vi "MMB SubVI.vi"(3 "Mode":T1(ring), 4 "Array Size":T2={"Width"=60, "Height"=17}, 5 "LED Off Color":u32(colorbox), 6 "LED Size":T2={"Width"=17, "Height"=17}, 7 "LED On Color":u32(colorbox)=4914962, 8 "Repeat/Hold":u64=1 min=1 step=1, 9 "Delay":u32(knob)=50 scale=0.0..1000.0, 10 "Message":string="The Quick Brown Fox Jumped Over the Lazy Dog", 11 "Config Path":path=path "c:/Ed's Files/LabVIEW Files/Moving Message Board/mmb.ini") -> ()   [LabVIEW 2010]
doc: "INTRODUCTION:\nThis program is a subVI implementation of the Moving Message Board program. It simulates a moving message board made up of an array of LED's or lights. It has multiple modes of operation.\n\nREQUIREMENTS:\nThe calling VI should pass the following inputs to it: the path of the configuration file, a string with the message to be displayed, an integer with the delay time, an integer with the repeat or hold value, and an enum with the operating mode.\n\nOPTIONAL:\nThe following can be passed if desired, but this is not required: a cluster with the \"on\" color of the LED's in the display, a cluster with the \"off\" color of the LED's in the display, a cluster containing the LED width and height, and a cluster containing the display size width and height (based on number of LED's in the array)."
uses:
  <vilib>/Utility/miscctls.llb/LVBoundsTypeDef.ctl
  <vilib>/Utility/miscctls.llb/LVPointTypeDef.ctl
  <vilib>/Utility/config.llb/Read Key (I32).vi
  <userlib>/_OpenG.lib/array/array.llb/Reorder 2D Array2 (Boolean)__ogtk.vi
  <vilib>/Utility/config.llb/NI_LVConfig.lvlib
panel:
  out "Array":bool[][](array[boolean])
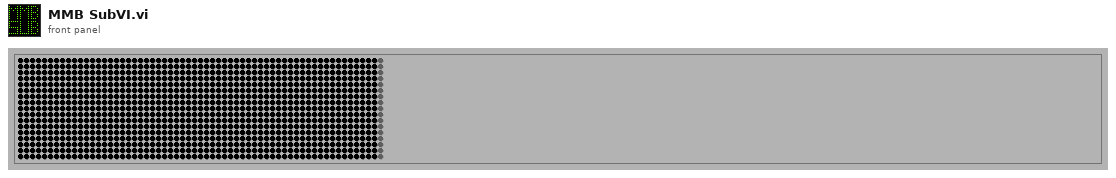
[diagram p1: front panel]
types:
  T1 = enum16{"Scrolling Message (0)", "Non-Scrolling Message (1)", "Fade In (2)", "Fade Out (3)", "Blink (4)", "Fly Up (5)", "Fall Down (6)", "Dissolve In (7)", "Dissolve Out (8)", "Random Pattern (9)"}
  T2 = typedef "LVBoundsTypeDef.ctl" = cluster{"Width":u32, "Height":u32}
  T3 = typedef "LVPointTypeDef.ctl" = cluster{"Horizontal":i16, "Vertical":i16}
  T4 = cluster{"LED Off Color":u32, "LED Off Color":u32}
  T5 = cluster{"LED On Color":u32, "LED On Color":u32}[]
  T6 = typedef "NI_LVConfig.lvlib/Config Data RefNum.ctl" = refnum<k1>
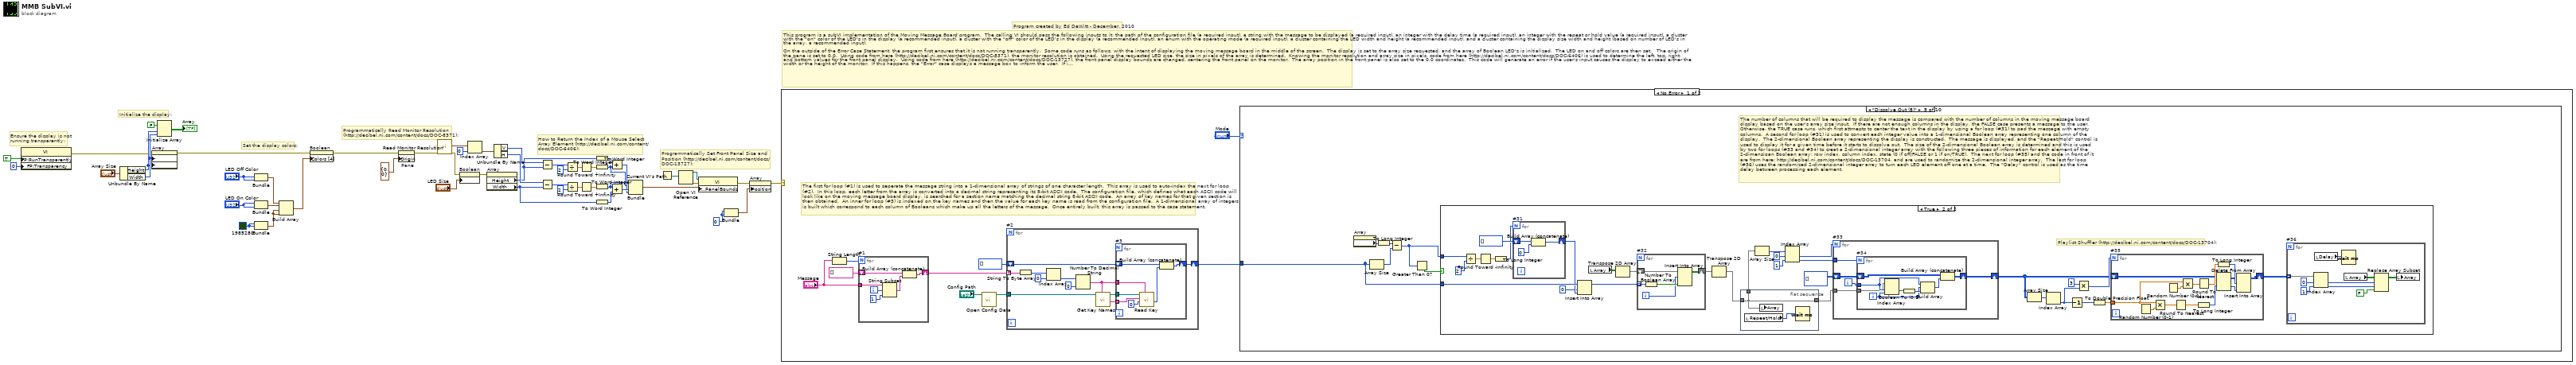
[diagram p0: block diagram]
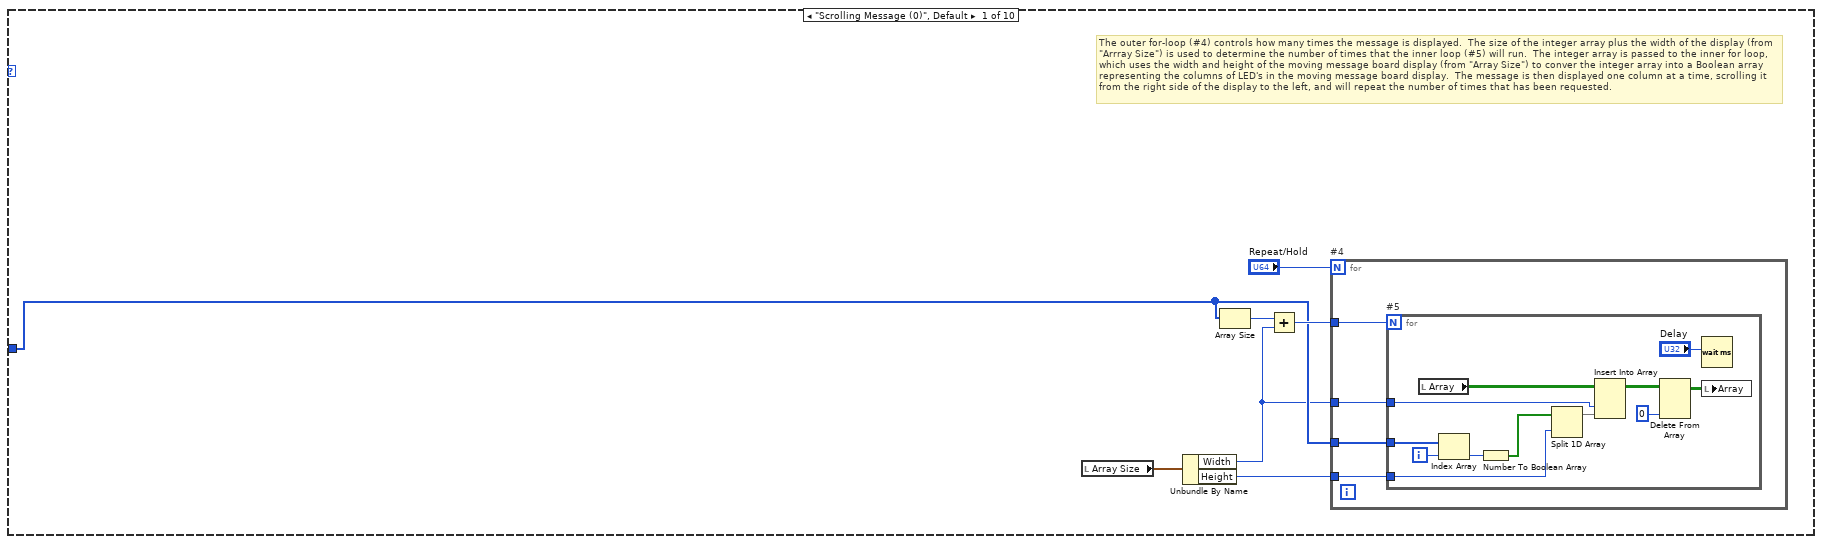
[diagram p2: hidden frame]
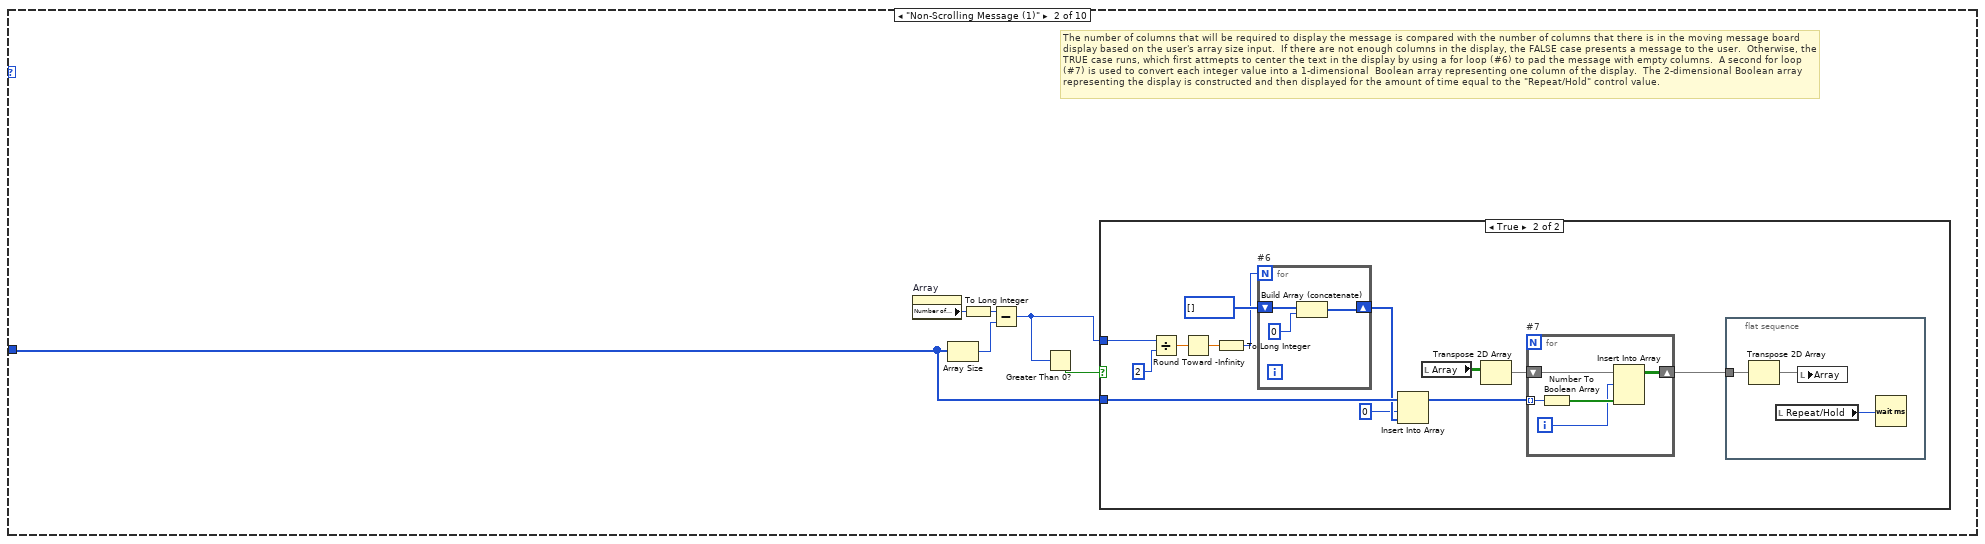
[diagram p3: hidden frame]
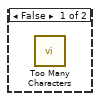
[diagram p4: hidden frame]
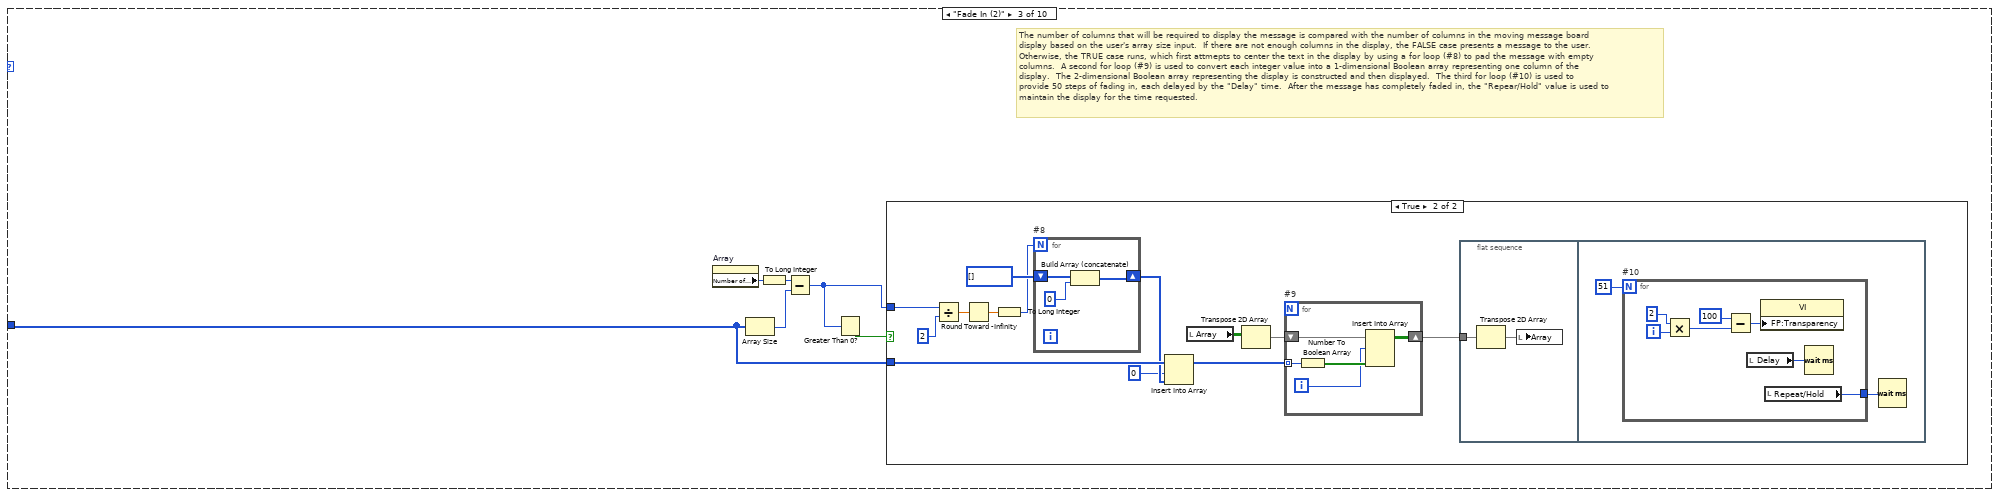
[diagram p5: hidden frame]
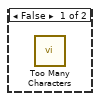
[diagram p6: hidden frame]
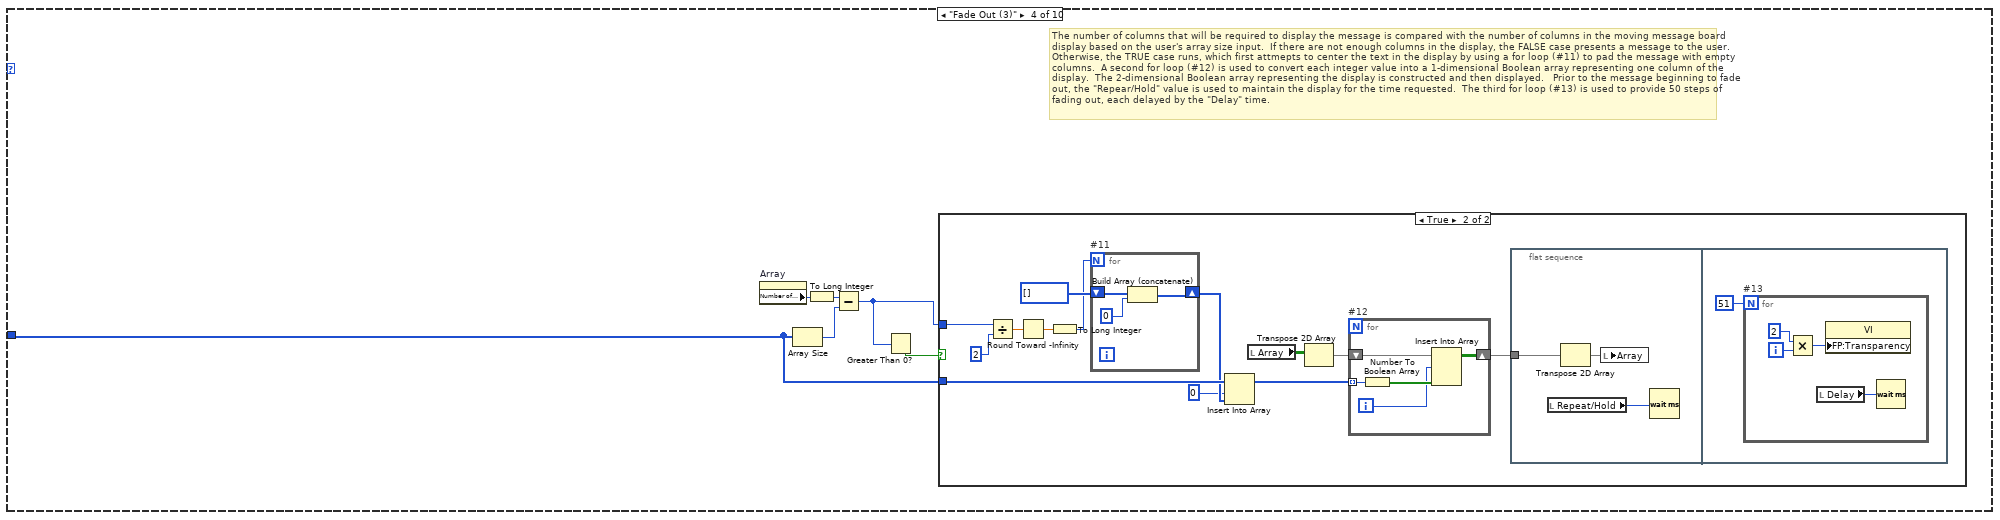
[diagram p7: hidden frame]
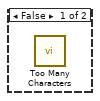
[diagram p8: hidden frame]
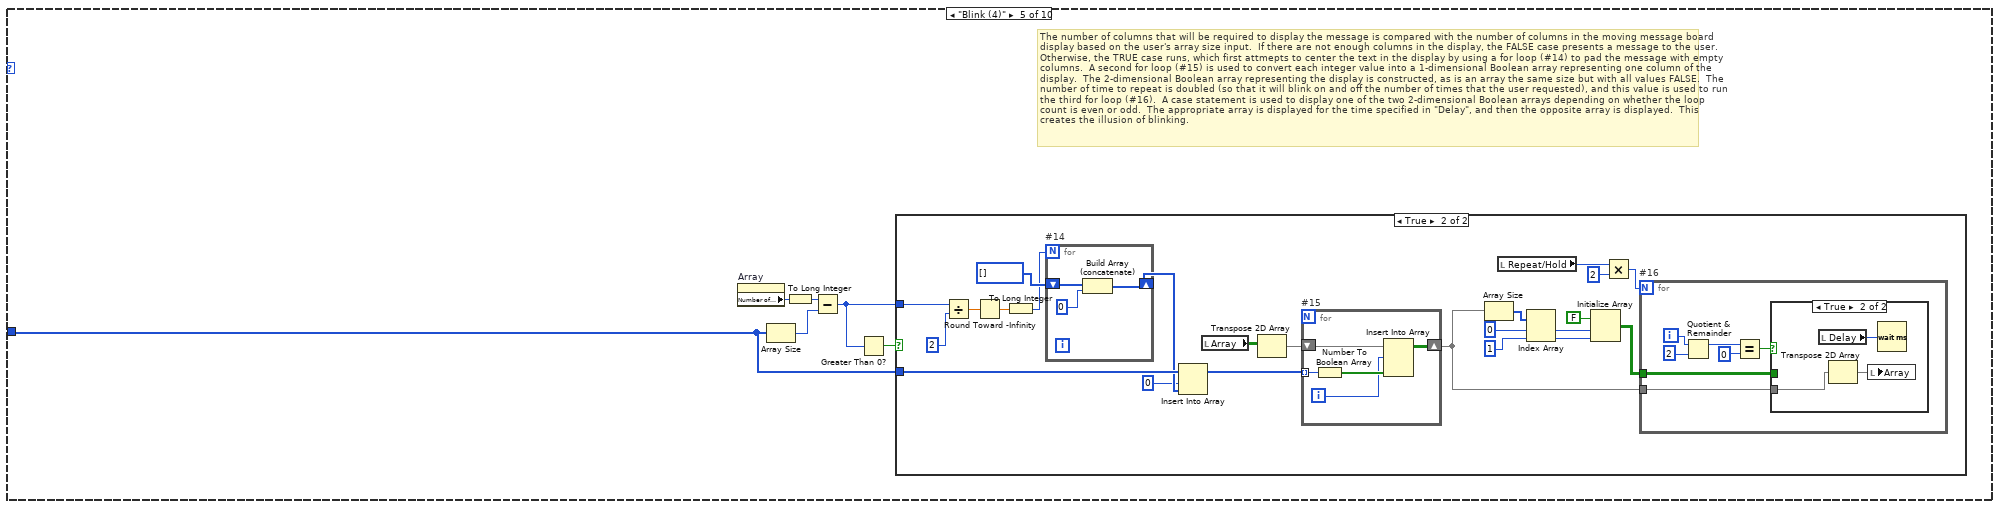
[diagram p9: hidden frame]
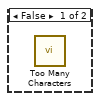
[diagram p10: hidden frame]
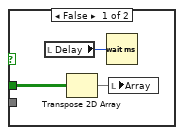
[diagram p11: hidden frame]
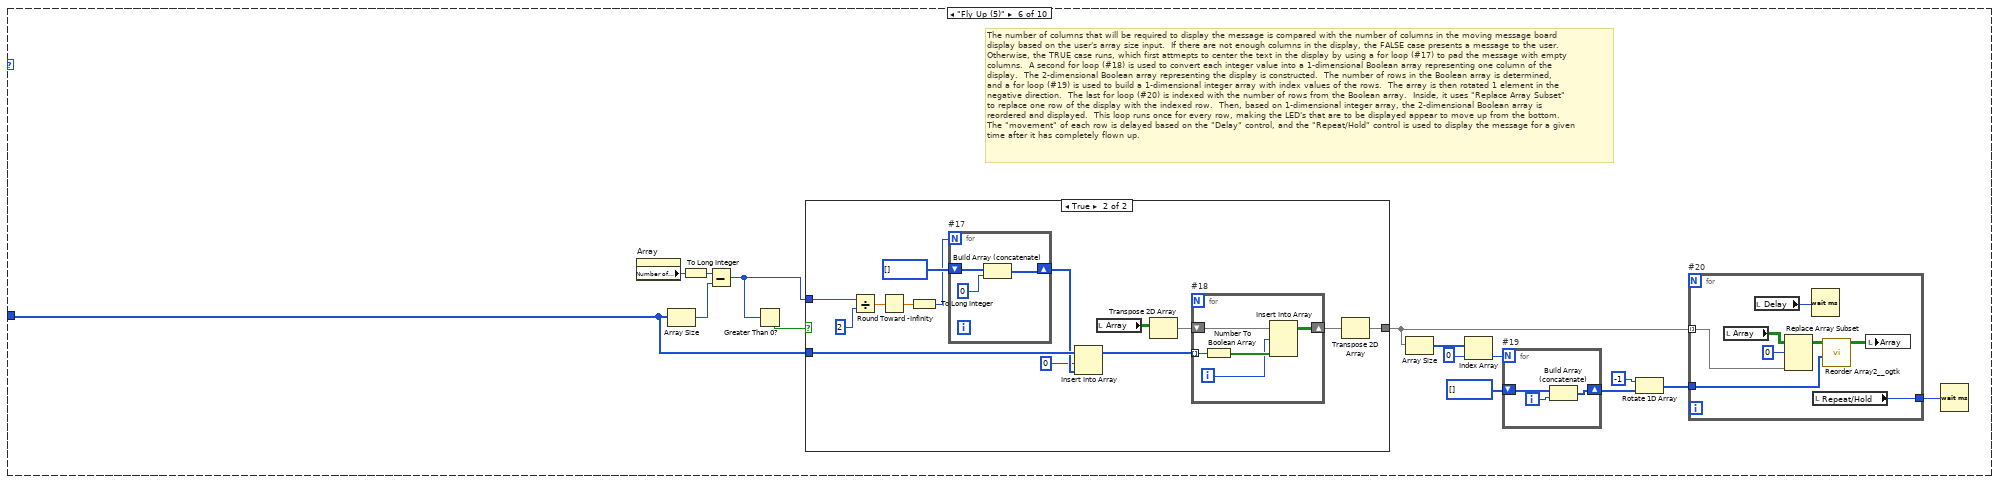
[diagram p12: hidden frame]
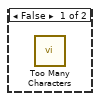
[diagram p13: hidden frame]
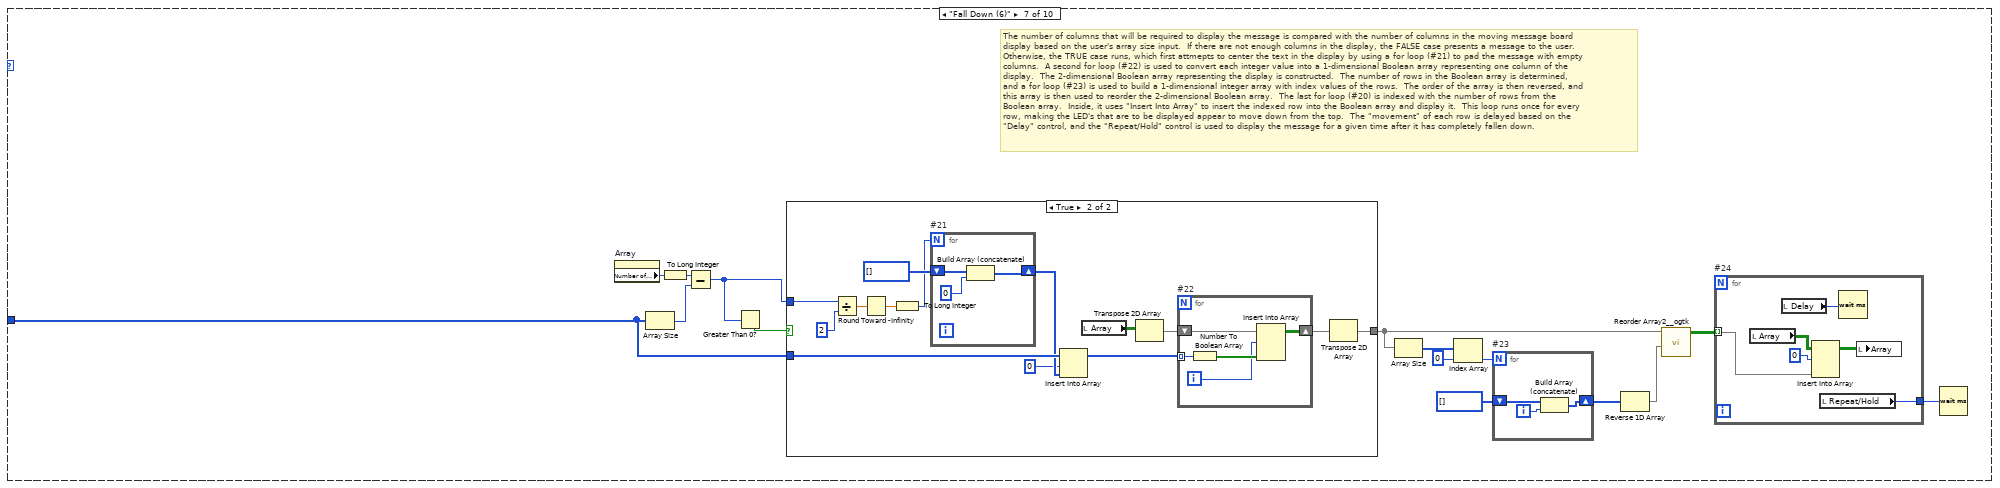
[diagram p14: hidden frame]
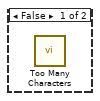
[diagram p15: hidden frame]
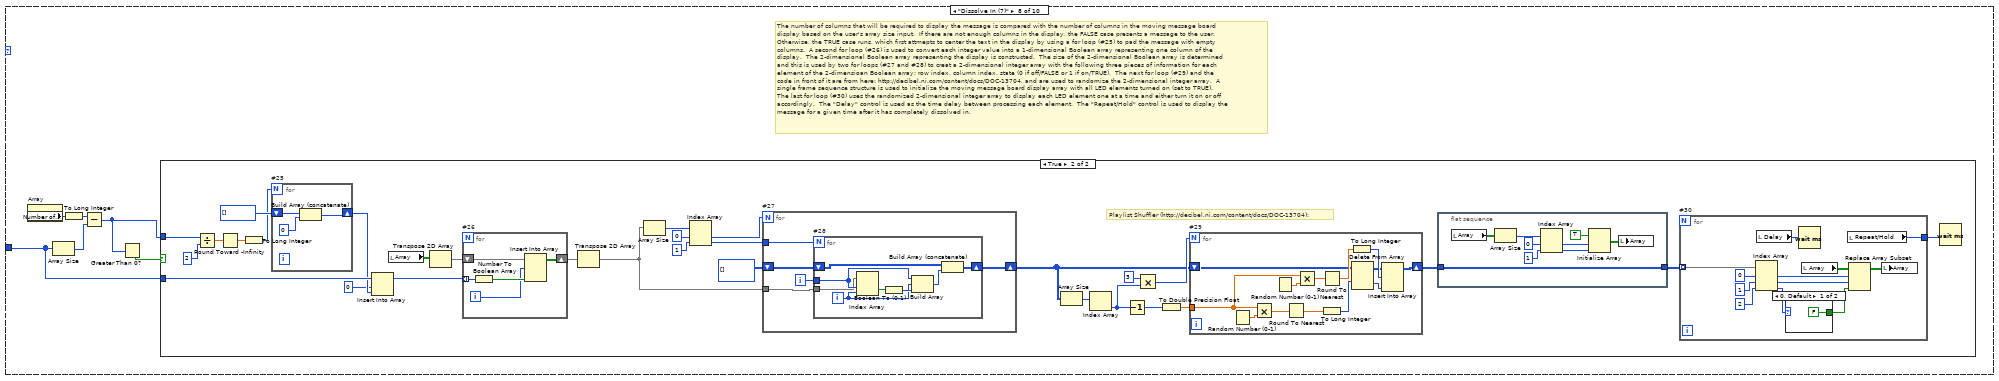
[diagram p16: hidden frame]
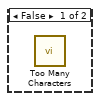
[diagram p17: hidden frame]
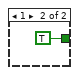
[diagram p18: hidden frame]
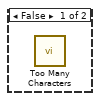
[diagram p19: hidden frame]
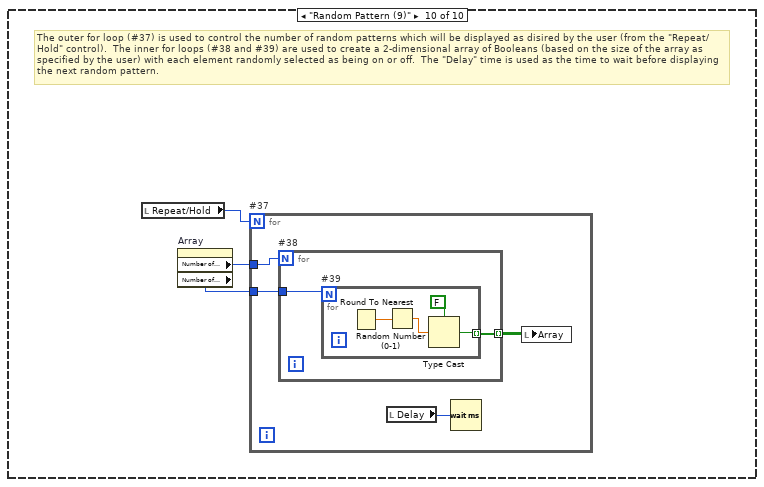
[diagram p20: hidden frame]
diagram:
  w15 = u32 0 ("y")
  w49 = u32 1985280
  # "This program is a subVI implementation of the Moving Message Board program.  The calling VI should pass the following inputs to it: the path of the configuration file (a required input), a string with the message to be displayed (a required input), an integer with the delay time (a required input), an integer with the repeat or hold value (a required input), a cluster with the \"on\" color of the LED's in the display (a recommended input), a cluster with the \"off\" color of the LED's in the display (a recommended input), an enum with the operating mode (a required input), a cluster containing the LED width and height (a recommended input), and a cluster containing the display size width and height (based on number of LED's in the array, a recommended input).\n\nOn the outside of the Error Case Statement, the program first ensures that it is not running transparently.  Some code runs as follows, with the intent of displaying the moving message board in the middle of the screen.  The display is set to the array size requested, and the array of Boolean LED's is initialized.  The LED on and off colors are then set.   The origin of the pane is set to 0,0.  Using code from here (http://decibel.ni.com/content/docs/DOC-8371), the monitor resolution is obtained.  Using the requested LED size, the size in pixels of the array is determined.  Knowing the monitor resolution and array size in pixels, code from here (http://decibel.ni.com/content/docs/DOC-6406) is used to determine the left, top, right, and bottom values for the front panel display.  Using code from here (http://decibel.ni.com/content/docs/DOC-13727), the front panel display bounds are changed, centering the front panel on the monitor.  The array position in the front panel is also set to the 0,0 coordinates.  This code will generate an error if the user's input causes the display to exceed either the width or the height of the monitor.  If this happens, the \"Error\" case displays a message box to inform the user.  If it doesn't happen then the \"No Error\" case runs."
  # "Initialize the display:"
  # "Ensure the display is not running transparently:"
  # "Programmatically Set Front Panel Size and Position (http://decibel.ni.com/content/docs/DOC-13727):"
  # "How to Return the Index of a Mouse Select Array Element (http://decibel.ni.com/content/docs/DOC-6406):"
  # "Programmatically Read Monitor Resolution\n(http://decibel.ni.com/content/docs/DOC-8371):"
  # "Set the display colors:"
  # "Program created by Ed DeWitt - December, 2010"
  n1 = property class="VI"("FP:RunTransparently"=TRUE ("Front Panel Window:Run VI Transparently"), "FP:Transparency"=u8 0 ("Front Panel Window:Transparency")) -> (error out=w6:errorcluster)  [unwired: 2 in, 1 out]
  n2 = Unbundle By Name("Array Size") -> ("Height"=w10:u32, "Width"=w11:u32)
  n3 = property on="Array" class="Arr (strict)"(error in=w6, "Number of Columns"=w11, "Number of Rows"=w10) -> (error out=w5:errorcluster)  [unwired: 1 in, 1 out]
  n4 = Initialize Array(FALSE, w10, w11) -> (→"Array":bool[][])
  n5 = Bundle("LED Off Color"="LED Off Color", "LED Off Color"="LED Off Color") -> (w51:T4)  [unwired: 1 out]
  n6 = Bundle("LED On Color"="LED On Color", "LED On Color"="LED On Color") -> (w45:cluster{"LED On Color":u32, "LED On Color":u32})  [unwired: 1 out]
  n7 = Bundle(w49, w49) -> (w46:cluster{u32, u32})  [unwired: 1 out]
  n8 = Build Array(w51, w45, w46, w46) -> (w48:T5)
  n9 = property on="Boolean" class="Bool (strict)"(error in=w5, "Colors [4]"=w48) -> (error out=w7:errorcluster)  [unwired: 1 in, 1 out]
  n10 = property on="Pane" class="Pane"(error in=w7, "Origin"=T3 {"Horizontal"=0, "Vertical"=0}) -> (error out=w2:errorcluster)  [unwired: 1 in, 1 out]
  n11 = call "Read Monitor Resolution.vi"("error in (no error)"=w2) -> ("error out"=w1:errorcluster, "Monitor Resolution"=w44:cluster{"V":i16, "H":i16}[])  [unwired: 8 in, 1 out]
  n12 = property on="Boolean" class="Bool (strict)"(error in=w1, "Button Size"="LED Size") -> (error out=w25:errorcluster)  [unwired: 1 in, 1 out]
  n13 = Index Array(array=w44, index=0) -> (element=w43:cluster{"V":i16, "H":i16})
  n14 = property on="Array" class="Arr (strict)"(error in=w25) -> ("Height"=w31:u32, "Width"=w34:u32)  [unwired: 1 in, 2 out]
  n15 = Unbundle By Name(w43) -> ("V"=w41:i16, "H"=w36:i16)
  n16 = Subtract(x=w41, y=w31) -> (x-y=w40:u32)
  n17 = Subtract(x=w36, y=w34) -> (x-y=w37:u32)
  n18 = Divide(x=w40, y=u32 2) -> (x/y=w32:dbl)
  n19 = Divide(x=w37, y=u32 2) -> (x/y=w35:dbl)
  n20 = Round Toward +Infinity(x=w32) -> (ceil(x): smallest int >= x=w28:dbl)
  n21 = Round Toward +Infinity(x=w35) -> (ceil(x): smallest int >= x=w29:dbl)
  n22 = To Word Integer(number=w31) -> (16bit integer=w26:i16)
  n23 = To Word Integer(number=w28) -> (16bit integer=w22:i16)
  n24 = To Word Integer(number=w29) -> (16bit integer=w23:i16)
  n25 = To Word Integer(number=w34) -> (16bit integer=w27:i16)
  n26 = Add(x=w26, y=w22) -> (x+y=w30:i16)
  n27 = Add(x=w23, y=w27) -> (x+y=w33:i16)
  n28 = Bundle(w23, w22, w33, w30) -> (w17:cluster{i16, i16, i16, i16})  [unwired: 1 in]
  n29 = Current VI's Path() -> (path=w20:path)
  n30 = Open VI Reference(vi path=w20) -> (vi reference=w18:refnum<vi>, error out=w19:errorcluster)  [unwired: 5 in]
  n31 = property class="VI"(reference=w18, error in=w19, "Front Panel.PanelBounds"=w17) -> (error out=w14:errorcluster)  [unwired: 1 out]
  n32 = Bundle("y"=w15, "y"=w15) -> (w16:cluster{"y":u32, "y":u32})  [unwired: 1 in]
  n33 = property on="Array" class="Arr (strict)"(error in=w14, "Position"=w16) -> (error out=w13:errorcluster)  [unwired: 1 in, 1 out]
  n34 = case shown="No Error" w13 {
    frame No Error {
      # "The first for loop (#1) is used to seperate the message string into a 1-dimensional array of strings of one character length.  This array is used to auto-index the next for loop (#2).  In this loop, each letter from the array is converted into a decimal string representing its 8-bit ASCII code.  The configuration file, which defines what each ASCII code will look like on the moving message board display, is searched for a section name matching the decimal string 8-bit ASCII code.  An array of key names for that given section is then obtained.  An inner for loop (#3) is indexed on the key names and then the value for each key name is read from the configuration file.  A 1-dimensional array of integers is built which correspond to each column of Booleans which make up all the letters of the message.  Once entirely built, this array is passed to the case statement."
      n35 = String Length(string="Message") -> (length=w54:i32)
      n36 = for "#1" {
        N: w54 -> [_]
        tunnel: "Message" -> [w66]
        shift-right: [w63] -> w53
        shift-left: string[] [] -> [w62]
        i -> [w65]
        n37 = String Subset(string=w66, offset (0)=w65, length (rest)=1 ("length (rest)")) -> (substring=w61:string)
        n38 = Build Array (concatenate)(w62, w61) -> (w63:string[])
      }
      n39 = call <vilib>:"Open Config Data.vi"("configuration file path"="Config Path") -> ("refnum"=w57:T6)  [unwired: 8 in, 2 out]
      n40 = for "#2" {
        tunnel: w57 -> [w77]
        tunnel: w53 -> [w68] mode=indexing
        shift-right: [w74] -> w52
        shift-left: i32[] [] -> [w73]
        n41 = String To Byte Array(string=w68) -> (unsigned byte array=w69:u8[])
        n42 = Index Array(array=w69, index=0) -> (element=w71:u8)
        n43 = Number To Decimal String(number=w71, width (-)=i16 0) -> (decimal integer string=w67:string)
        n44 = call <vilib>:"Get Key Names.vi"("section"=w67, "refnum"=w77) -> ("key names"=w76:string[], "refnum out"=w75:T6)  [unwired: 1 in, 7 out]
        n45 = for "#3" {
          tunnel: w76 -> [w83] mode=indexing
          tunnel: w75 -> [w82]
          shift-right: [w78] -> w74
          shift-left: w73 -> [w79]
          tunnel: w67 -> [w84]
          n46 = call-poly <vilib>:"Read Key.vi"("section"=w84, "default value"=0, "key"=w83, "refnum"=w82) -> ("value"=w81:i32)  [unwired: 1 in, 6 out]
          n47 = Build Array (concatenate)(w79, w81) -> (w78:i32[])
        }
      }
      n48 = case shown="\"Dissolve Out (8)\"" "Mode" {
        tunnel: w52 -> [w87 w108 w138 w176 w211 w261 w309 w355 w448 _]
        frame "Scrolling Message (0)", Default {
          # "The outer for-loop (#4) controls how many times the message is displayed.  The size of the integer array plus the width of the display (from \"Arrray Size\") is used to determine the number of times that the inner loop (#5) will run.  The integer array is passed to the inner for loop, which uses the width and height of the moving message board display (from \"Array Size\") to conver the integer array into a Boolean array representing the columns of LED's in the moving message board display.  The message is then displayed one column at a time, scrolling it from the right side of the display to the left, and will repeat the number of times that has been requested."
          n49 = local read "Array Size"() -> (w89:T2)
          n50 = Unbundle By Name(w89) -> ("Width"=w86:u32, "Height"=w85:u32)
          n51 = Array Size(array=w87) -> (size(s)=w90:i32)
          n52 = Add(x=w90, y=w86) -> (x+y=w88:u32)
          n53 = for "#4" {
            N: "Repeat/Hold" -> [_]
            tunnel: w88 -> [w95]
            tunnel: w87 -> [w94]
            tunnel: w86 -> [w93]
            tunnel: w85 -> [w92]
            n54 = for "#5" {
              N: w95 -> [_]
              tunnel: w94 -> [w106]
              tunnel: w93 -> [w97]
              tunnel: w92 -> [w96]
              i -> [w105]
              n55 = local read "Array"() -> (w107:bool[][])
              n56 = Index Array(array=w106, index=w105) -> (element=w104:i32)
              n57 = Number To Boolean Array(number=w104) -> (Boolean array=w100:bool[])
              n58 = Split 1D Array(array=w100, index=w96) -> (first subarray=w99:bool[])  [unwired: 1 out]
              n59 = Insert Into Array(array=w107, index (col)=w97, new element=w99) -> (w103:bool[][])  [unwired: 1 in]
              n60 = Delete From Array(array=w103, index (col)=0 ("disabled index (col)")) -> (array with subset deleted=w101:bool[][])  [unwired: 2 in, 1 out]
              n61 = Wait (ms)(milliseconds to wait="Delay") -> ()  [unwired: 1 out]
              n62 = local write "Array"(w101) -> ()
            }
          }
        }
        frame "Non-Scrolling Message (1)" {
          # "The number of columns that will be required to display the message is compared with the number of columns that there is in the moving message board display based on the user's array size input.  If there are not enough columns in the display, the FALSE case presents a message to the user.  Otherwise, the TRUE case runs, which first attmepts to center the text in the display by using a for loop (#6) to pad the message with empty columns.  A second for loop (#7) is used to convert each integer value into a 1-dimensional  Boolean array representing one column of the display.  The 2-dimensional Boolean array representing the display is constructed and then displayed for the amount of time equal to the \"Repeat/Hold\" control value."
          n63 = property on="Array" class="Arr (strict)"() -> ("Number of Columns"=w113:u32)  [unwired: 2 in, 2 out]
          n64 = Array Size(array=w108) -> (size(s)=w112:i32)
          n65 = To Long Integer(number=w113) -> (32bit integer=w109:i32)
          n66 = Subtract(x=w109, y=w112) -> (x-y=w110:i32)
          n67 = Greater Than 0?(x=w110) -> (x > 0?=w111:bool)
          n68 = case shown="True" w111 {
            tunnel: w110 -> [_ w126]
            tunnel: w108 -> [_ w124]
            frame False {
              n69 = call "Too Many Characters.vi"() -> ()  [unwired: 12 in]
            }
            frame True {
              n70 = Divide(x=w126, y=u32 2) -> (x/y=w123:dbl)
              n71 = Round Toward -Infinity(1:w123) -> (0:w122:dbl)
              n72 = To Long Integer(number=w122) -> (32bit integer=w120:i32)
              n73 = for "#6" {
                N: w120 -> [_]
                shift-right: [w135] -> w119
                shift-left: i32[] [] -> [w137]
                n74 = Build Array (concatenate)(w137, i16 0 ("width (-)")) -> (w135:i32[])
              }
              n75 = Insert Into Array(array=w124, index=0, new element=w119) -> (w115:i32[])
              n76 = local read "Array"() -> (w116:bool[][])
              n77 = Transpose 2D Array(2D array=w116) -> (transposed array=w114:bool[][])
              n78 = for "#7" {
                shift-right: [w133] -> w117
                shift-left: w114 -> [w132]
                tunnel: w115 -> [w131] mode=indexing
                i -> [w130]
                n79 = Number To Boolean Array(number=w131) -> (Boolean array=w134:bool[])
                n80 = Insert Into Array(array=w132, index (row)=w130, new element=w134) -> (w133:bool[][])  [unwired: 1 in]
              }
              n81 = flat-sequence {
                tunnel: w117 -> [w129]
                frame #0 {
                  n82 = Transpose 2D Array(2D array=w129) -> (transposed array=w128:bool[][])
                  n83 = local read "Repeat/Hold"() -> (w127:u64)
                  n84 = local write "Array"(w128) -> ()
                  n85 = Wait (ms)(milliseconds to wait=w127) -> ()  [unwired: 1 out]
                }
              }
            }
          }
        }
        frame "Fade In (2)" {
          # "The number of columns that will be required to display the message is compared with the number of columns in the moving message board display based on the user's array size input.  If there are not enough columns in the display, the FALSE case presents a message to the user.  Otherwise, the TRUE case runs, which first attmepts to center the text in the display by using a for loop (#8) to pad the message with empty columns.  A second for loop (#9) is used to convert each integer value into a 1-dimensional Boolean array representing one column of the display.  The 2-dimensional Boolean array representing the display is constructed and then displayed.  The third for loop (#10) is used to provide 50 steps of fading in, each delayed by the \"Delay\" time.  After the message has completely faded in, the \"Repear/Hold\" value is used to maintain the display for the time requested."
          n86 = property on="Array" class="Arr (strict)"() -> ("Number of Columns"=w143:u32)  [unwired: 2 in, 2 out]
          n87 = Array Size(array=w138) -> (size(s)=w142:i32)
          n88 = To Long Integer(number=w143) -> (32bit integer=w139:i32)
          n89 = Subtract(x=w139, y=w142) -> (x-y=w140:i32)
          n90 = Greater Than 0?(x=w140) -> (x > 0?=w141:bool)
          n91 = case shown="True" w141 {
            tunnel: w140 -> [_ w156]
            tunnel: w138 -> [_ w154]
            frame False {
              n92 = call "Too Many Characters.vi"() -> ()  [unwired: 12 in]
            }
            frame True {
              n93 = Divide(x=w156, y=u32 2) -> (x/y=w153:dbl)
              n94 = Round Toward -Infinity(1:w153) -> (0:w152:dbl)
              n95 = To Long Integer(number=w152) -> (32bit integer=w150:i32)
              n96 = for "#8" {
                N: w150 -> [_]
                shift-right: [w173] -> w149
                shift-left: i32[] [] -> [w175]
                n97 = Build Array (concatenate)(w175, i16 0 ("width (-)")) -> (w173:i32[])
              }
              n98 = Insert Into Array(array=w154, index=0, new element=w149) -> (w145:i32[])
              n99 = local read "Array"() -> (w146:bool[][])
              n100 = Transpose 2D Array(2D array=w146) -> (transposed array=w144:bool[][])
              n101 = for "#9" {
                shift-right: [w171] -> w147
                shift-left: w144 -> [w170]
                tunnel: w145 -> [w169] mode=indexing
                i -> [w168]
                n102 = Number To Boolean Array(number=w169) -> (Boolean array=w172:bool[])
                n103 = Insert Into Array(array=w170, index (row)=w168, new element=w172) -> (w171:bool[][])  [unwired: 1 in]
              }
              n104 = flat-sequence {
                tunnel: w147 -> [w158]
                frame #0 {
                  n105 = Transpose 2D Array(2D array=w158) -> (transposed array=w157:bool[][])
                  n106 = local write "Array"(w157) -> ()
                }
                frame #1 {
                  n107 = for "#10" {
                    N: 51 -> [_]
                    tunnel: [w161] -> w159
                    i -> [w164]
                    n108 = Multiply(x=2, y=w164) -> (x*y=w162:i32)
                    n109 = Subtract(x=100, y=w162) -> (x-y=w166:i32)
                    n110 = local read "Delay"() -> (w167:u32)
                    n111 = property class="VI"("FP:Transparency"=w166) -> ()  [unwired: 2 in, 2 out]
                    n112 = local read "Repeat/Hold"() -> (w161:u64)
                    n113 = Wait (ms)(milliseconds to wait=w167) -> ()  [unwired: 1 out]
                  }
                  n114 = Wait (ms)(milliseconds to wait=w159) -> ()  [unwired: 1 out]
                }
              }
            }
          }
        }
        frame "Fade Out (3)" {
          # "The number of columns that will be required to display the message is compared with the number of columns in the moving message board display based on the user's array size input.  If there are not enough columns in the display, the FALSE case presents a message to the user.  Otherwise, the TRUE case runs, which first attmepts to center the text in the display by using a for loop (#11) to pad the message with empty columns.  A second for loop (#12) is used to convert each integer value into a 1-dimensional Boolean array representing one column of the display.  The 2-dimensional Boolean array representing the display is constructed and then displayed.   Prior to the message beginning to fade out, the \"Repear/Hold\" value is used to maintain the display for the time requested.  The third for loop (#13) is used to provide 50 steps of fading out, each delayed by the \"Delay\" time."
          n115 = property on="Array" class="Arr (strict)"() -> ("Number of Columns"=w181:u32)  [unwired: 2 in, 2 out]
          n116 = Array Size(array=w176) -> (size(s)=w180:i32)
          n117 = To Long Integer(number=w181) -> (32bit integer=w177:i32)
          n118 = Subtract(x=w177, y=w180) -> (x-y=w178:i32)
          n119 = Greater Than 0?(x=w178) -> (x > 0?=w179:bool)
          n120 = case shown="True" w179 {
            tunnel: w178 -> [_ w194]
            tunnel: w176 -> [_ w192]
            frame False {
              n121 = call "Too Many Characters.vi"() -> ()  [unwired: 12 in]
            }
            frame True {
              n122 = Divide(x=w194, y=u32 2) -> (x/y=w191:dbl)
              n123 = Round Toward -Infinity(1:w191) -> (0:w190:dbl)
              n124 = To Long Integer(number=w190) -> (32bit integer=w188:i32)
              n125 = for "#11" {
                N: w188 -> [_]
                shift-right: [w208] -> w187
                shift-left: i32[] [] -> [w210]
                n126 = Build Array (concatenate)(w210, i16 0 ("width (-)")) -> (w208:i32[])
              }
              n127 = Insert Into Array(array=w192, index=0, new element=w187) -> (w183:i32[])
              n128 = local read "Array"() -> (w184:bool[][])
              n129 = Transpose 2D Array(2D array=w184) -> (transposed array=w182:bool[][])
              n130 = for "#12" {
                shift-right: [w206] -> w185
                shift-left: w182 -> [w205]
                tunnel: w183 -> [w204] mode=indexing
                i -> [w203]
                n131 = Number To Boolean Array(number=w204) -> (Boolean array=w207:bool[])
                n132 = Insert Into Array(array=w205, index (row)=w203, new element=w207) -> (w206:bool[][])  [unwired: 1 in]
              }
              n133 = flat-sequence {
                tunnel: w185 -> [w197]
                frame #0 {
                  n134 = local read "Repeat/Hold"() -> (w195:u64)
                  n135 = Transpose 2D Array(2D array=w197) -> (transposed array=w196:bool[][])
                  n136 = local write "Array"(w196) -> ()
                  n137 = Wait (ms)(milliseconds to wait=w195) -> ()  [unwired: 1 out]
                }
                frame #1 {
                  n138 = for "#13" {
                    N: 51 -> [_]
                    i -> [w201]
                    n139 = Multiply(x=2, y=w201) -> (x*y=w199:i32)
                    n140 = local read "Delay"() -> (w202:u32)
                    n141 = property class="VI"("FP:Transparency"=w199) -> ()  [unwired: 2 in, 2 out]
                    n142 = Wait (ms)(milliseconds to wait=w202) -> ()  [unwired: 1 out]
                  }
                }
              }
            }
          }
        }
        frame "Blink (4)" {
          # "The number of columns that will be required to display the message is compared with the number of columns in the moving message board display based on the user's array size input.  If there are not enough columns in the display, the FALSE case presents a message to the user.  Otherwise, the TRUE case runs, which first attmepts to center the text in the display by using a for loop (#14) to pad the message with empty columns.  A second for loop (#15) is used to convert each integer value into a 1-dimensional Boolean array representing one column of the display.  The 2-dimensional Boolean array representing the display is constructed, as is an array the same size but with all values FALSE.  The number of time to repeat is doubled (so that it will blink on and off the number of times that the user requested), and this value is used to run the third for loop (#16).  A case statement is used to display one of the two 2-dimensional Boolean arrays depending on whether the loop count is even or odd.  The appropriate array is displayed for the time specified in \"Delay\", and then the opposite array is displayed.  This creates the illusion of blinking."
          n143 = property on="Array" class="Arr (strict)"() -> ("Number of Columns"=w216:u32)  [unwired: 2 in, 2 out]
          n144 = Array Size(array=w211) -> (size(s)=w215:i32)
          n145 = To Long Integer(number=w216) -> (32bit integer=w212:i32)
          n146 = Subtract(x=w212, y=w215) -> (x-y=w213:i32)
          n147 = Greater Than 0?(x=w213) -> (x > 0?=w214:bool)
          n148 = case shown="True" w214 {
            tunnel: w213 -> [_ w239]
            tunnel: w211 -> [_ w237]
            frame False {
              n149 = call "Too Many Characters.vi"() -> ()  [unwired: 12 in]
            }
            frame True {
              n150 = Divide(x=w239, y=u32 2) -> (x/y=w236:dbl)
              n151 = Round Toward -Infinity(1:w236) -> (0:w235:dbl)
              n152 = To Long Integer(number=w235) -> (32bit integer=w233:i32)
              n153 = for "#14" {
                N: w233 -> [_]
                shift-right: [w258] -> w232
                shift-left: i32[] [] -> [w260]
                n154 = Build Array (concatenate)(w260, i16 0 ("width (-)")) -> (w258:i32[])
              }
              n155 = Insert Into Array(array=w237, index=0, new element=w232) -> (w229:i32[])
              n156 = local read "Array"() -> (w230:bool[][])
              n157 = Transpose 2D Array(2D array=w230) -> (transposed array=w228:bool[][])
              n158 = for "#15" {
                shift-right: [w256] -> w224
                shift-left: w228 -> [w255]
                tunnel: w229 -> [w254] mode=indexing
                i -> [w253]
                n159 = Number To Boolean Array(number=w254) -> (Boolean array=w257:bool[])
                n160 = Insert Into Array(array=w255, index (row)=w253, new element=w257) -> (w256:bool[][])  [unwired: 1 in]
              }
              n161 = Array Size(array=w224) -> (size(s)=w223:i32[])
              n162 = local read "Repeat/Hold"() -> (w227:u64)
              n163 = Index Array(array=w223, index #1=0 ("index"), index #2=1 ("index")) -> (element #1=w220:i32, element #2=w219:i32)
              n164 = Initialize Array(FALSE, w220, w219) -> (w217:bool[][])
              n165 = Multiply(x=w227, y=2 ("index")) -> (x*y=w225:u64)
              n166 = for "#16" {
                N: w225 -> [_]
                tunnel: w224 -> [w241]
                tunnel: w217 -> [w240]
                i -> [w246]
                n167 = Quotient & Remainder(x=w246, y=2 ("index")) -> (x-y*floor(x/y)=w244:i32)  [unwired: 1 out]
                n168 = Equal?(x=w244, y=0 ("index")) -> (x = y?=w242:bool)
                n169 = case shown="True" w242 {
                  tunnel: w241 -> [_ w251]
                  tunnel: w240 -> [w247 _]
                  frame False {
                    n170 = local read "Delay"() -> (w249:u32)
                    n171 = Transpose 2D Array(2D array=w247) -> (transposed array=w248:bool[][])
                    n172 = Wait (ms)(milliseconds to wait=w249) -> ()  [unwired: 1 out]
                    n173 = local write "Array"(w248) -> ()
                  }
                  frame True {
                    n174 = local read "Delay"() -> (w250:u32)
                    n175 = Transpose 2D Array(2D array=w251) -> (transposed array=w252:bool[][])
                    n176 = local write "Array"(w252) -> ()
                    n177 = Wait (ms)(milliseconds to wait=w250) -> ()  [unwired: 1 out]
                  }
                }
              }
            }
          }
        }
        frame "Fly Up (5)" {
          # "The number of columns that will be required to display the message is compared with the number of columns in the moving message board display based on the user's array size input.  If there are not enough columns in the display, the FALSE case presents a message to the user.  Otherwise, the TRUE case runs, which first attmepts to center the text in the display by using a for loop (#17) to pad the message with empty columns.  A second for loop (#18) is used to convert each integer value into a 1-dimensional Boolean array representing one column of the display.  The 2-dimensional Boolean array representing the display is constructed.  The number of rows in the Boolean array is determined, and a for loop (#19) is used to build a 1-dimensional integer array with index values of the rows.  The array is then rotated 1 element in the negative direction.  The last for loop (#20) is indexed with the number of rows from the Boolean array.  Inside, it uses \"Replace Array Subset\" to replace one row of the display with the indexed row.  Then, based on 1-dimensional integer array, the 2-dimensional Boolean array is reordered and displayed.  This loop runs once for every row, making the LED's that are to be displayed appear to move up from the bottom.  The \"movement\" of each row is delayed based on the \"Delay\" control, and the \"Repeat/Hold\" control is used to display the message for a given time after it has completely flown up."
          n178 = property on="Array" class="Arr (strict)"() -> ("Number of Columns"=w275:u32)  [unwired: 2 in, 2 out]
          n179 = Array Size(array=w261) -> (size(s)=w274:i32)
          n180 = To Long Integer(number=w275) -> (32bit integer=w271:i32)
          n181 = Subtract(x=w271, y=w274) -> (x-y=w272:i32)
          n182 = Greater Than 0?(x=w272) -> (x > 0?=w273:bool)
          n183 = case shown="True" w273 {
            tunnel: w272 -> [_ w300]
            tunnel: w261 -> [_ w298]
            tunnel: [_ w287] -> w263
            frame False {
              n184 = call "Too Many Characters.vi"() -> ()  [unwired: 12 in]
            }
            frame True {
              n185 = Divide(x=w300, y=u32 2) -> (x/y=w297:dbl)
              n186 = Round Toward -Infinity(1:w297) -> (0:w296:dbl)
              n187 = To Long Integer(number=w296) -> (32bit integer=w294:i32)
              n188 = for "#17" {
                N: w294 -> [_]
                shift-right: [w306] -> w293
                shift-left: i32[] [] -> [w308]
                n189 = Build Array (concatenate)(w308, i16 0 ("width (-)")) -> (w306:i32[])
              }
              n190 = Insert Into Array(array=w298, index=0, new element=w293) -> (w289:i32[])
              n191 = local read "Array"() -> (w290:bool[][])
              n192 = Transpose 2D Array(2D array=w290) -> (transposed array=w288:bool[][])
              n193 = for "#18" {
                shift-right: [w304] -> w291
                shift-left: w288 -> [w303]
                tunnel: w289 -> [w302] mode=indexing
                i -> [w301]
                n194 = Number To Boolean Array(number=w302) -> (Boolean array=w305:bool[])
                n195 = Insert Into Array(array=w303, index (row)=w301, new element=w305) -> (w304:bool[][])  [unwired: 1 in]
              }
              n196 = Transpose 2D Array(2D array=w291) -> (transposed array=w287:bool[][])
            }
          }
          n197 = Array Size(array=w263) -> (size(s)=w265:i32[])
          n198 = Index Array(array=w265, index=0) -> (element=w267:i32)
          n199 = for "#19" {
            N: w267 -> [_]
            shift-right: [w284] -> w269
            shift-left: i32[] [] -> [w286]
            i -> [w285]
            n200 = Build Array (concatenate)(w286, w285) -> (w284:i32[])
          }
          n201 = Rotate 1D Array(1:w269, 2:-1 ("n")) -> (0:w264:i32[])
          n202 = for "#20" {
            tunnel: w263 -> [w281] mode=indexing
            tunnel: w264 -> [w278]
            tunnel: [w276] -> w262
            n203 = local read "Array"() -> (w283:bool[][])
            n204 = local read "Delay"() -> (w277:u32)
            n205 = Replace Array Subset(array=w283, new element=w281, index (row)=0) -> (w280:bool[][])  [unwired: 1 in]
            n206 = Wait (ms)(milliseconds to wait=w277) -> ()  [unwired: 1 out]
            n207 = local read "Repeat/Hold"() -> (w276:u64)
            n208 = call-poly <userlib>:"Reorder Array2__ogtk.vi"("indices"=w278, "array"=w280) -> ("reordered array"=w279:bool[][])  [unwired: 9 in]
            n209 = local write "Array"(w279) -> ()
          }
          n210 = Wait (ms)(milliseconds to wait=w262) -> ()  [unwired: 1 out]
        }
        frame "Fall Down (6)" {
          # "The number of columns that will be required to display the message is compared with the number of columns in the moving message board display based on the user's array size input.  If there are not enough columns in the display, the FALSE case presents a message to the user.  Otherwise, the TRUE case runs, which first attmepts to center the text in the display by using a for loop (#21) to pad the message with empty columns.  A second for loop (#22) is used to convert each integer value into a 1-dimensional Boolean array representing one column of the display.  The 2-dimensional Boolean array representing the display is constructed.  The number of rows in the Boolean array is determined, and a for loop (#23) is used to build a 1-dimensional integer array with index values of the rows.  The order of the array is then reversed, and this array is then used to reorder the 2-dimensional Boolean array.  The last for loop (#20) is indexed with the number of rows from the Boolean array.  Inside, it uses \"Insert Into Array\" to insert the indexed row into the Boolean array and display it.  This loop runs once for every row, making the LED's that are to be displayed appear to move down from the top.  The \"movement\" of each row is delayed based on the \"Delay\" control, and the \"Repeat/Hold\" control is used to display the message for a given time after it has completely fallen down."
          n211 = property on="Array" class="Arr (strict)"() -> ("Number of Columns"=w323:u32)  [unwired: 2 in, 2 out]
          n212 = Array Size(array=w309) -> (size(s)=w322:i32)
          n213 = To Long Integer(number=w323) -> (32bit integer=w319:i32)
          n214 = Subtract(x=w319, y=w322) -> (x-y=w320:i32)
          n215 = Greater Than 0?(x=w320) -> (x > 0?=w321:bool)
          n216 = case shown="True" w321 {
            tunnel: w320 -> [_ w346]
            tunnel: w309 -> [_ w344]
            tunnel: [_ w333] -> w312
            frame False {
              n217 = call "Too Many Characters.vi"() -> ()  [unwired: 12 in]
            }
            frame True {
              n218 = Divide(x=w346, y=u32 2) -> (x/y=w343:dbl)
              n219 = Round Toward -Infinity(1:w343) -> (0:w342:dbl)
              n220 = To Long Integer(number=w342) -> (32bit integer=w340:i32)
              n221 = for "#21" {
                N: w340 -> [_]
                shift-right: [w352] -> w339
                shift-left: i32[] [] -> [w354]
                n222 = Build Array (concatenate)(w354, i16 0 ("width (-)")) -> (w352:i32[])
              }
              n223 = Insert Into Array(array=w344, index=0, new element=w339) -> (w335:i32[])
              n224 = local read "Array"() -> (w336:bool[][])
              n225 = Transpose 2D Array(2D array=w336) -> (transposed array=w334:bool[][])
              n226 = for "#22" {
                shift-right: [w350] -> w337
                shift-left: w334 -> [w349]
                tunnel: w335 -> [w348] mode=indexing
                i -> [w347]
                n227 = Number To Boolean Array(number=w348) -> (Boolean array=w351:bool[])
                n228 = Insert Into Array(array=w349, index (row)=w347, new element=w351) -> (w350:bool[][])  [unwired: 1 in]
              }
              n229 = Transpose 2D Array(2D array=w337) -> (transposed array=w333:bool[][])
            }
          }
          n230 = Array Size(array=w312) -> (size(s)=w315:i32[])
          n231 = Index Array(array=w315, index=0) -> (element=w317:i32)
          n232 = for "#23" {
            N: w317 -> [_]
            shift-right: [w330] -> w313
            shift-left: i32[] [] -> [w332]
            i -> [w331]
            n233 = Build Array (concatenate)(w332, w331) -> (w330:i32[])
          }
          n234 = Reverse 1D Array(array=w313) -> (reversed array=w311:i32[])
          n235 = call-poly <userlib>:"Reorder Array2__ogtk.vi"("indices"=w311, "array"=w312) -> ("reordered array"=w310:bool[][])  [unwired: 9 in]
          n236 = for "#24" {
            tunnel: w310 -> [w327] mode=indexing
            tunnel: [w325] -> w314
            n237 = local read "Array"() -> (w329:bool[][])
            n238 = local read "Delay"() -> (w326:u32)
            n239 = Insert Into Array(array=w329, index (row)=0, new element=w327) -> (w324:bool[][])  [unwired: 1 in]
            n240 = local read "Repeat/Hold"() -> (w325:u64)
            n241 = Wait (ms)(milliseconds to wait=w326) -> ()  [unwired: 1 out]
            n242 = local write "Array"(w324) -> ()
          }
          n243 = Wait (ms)(milliseconds to wait=w314) -> ()  [unwired: 1 out]
        }
        frame "Dissolve In (7)" {
          # "The number of columns that will be required to display the message is compared with the number of columns in the moving message board display based on the user's array size input.  If there are not enough columns in the display, the FALSE case presents a message to the user.  Otherwise, the TRUE case runs, which first attmepts to center the text in the display by using a for loop (#25) to pad the message with empty columns.  A second for loop (#26) is used to convert each integer value into a 1-dimensional Boolean array representing one column of the display.  The 2-dimensional Boolean array representing the display is constructed.  The size of the 2-dimensional Boolean array is determined and this is used by two for loops (#27 and #28) to creat a 2-dimensional integer array with the following three pieces of information for each element of the 2-dimensioan Boolean array: row index, column index, state (0 if off/FALSE or 1 if on/TRUE).  The next for loop (#29) and the code in front of it are from here: http://decibel.ni.com/content/docs/DOC-13704, and are used to randomize the 2-dimensional integer array.  A single frame sequence structure is used to initialize the moving message board display array with all LED elements turned on (set to TRUE).  The last for loop (#30) uses the randomized 2-dimensional integer array to display each LED element one at a time and either turn it on or off accordingly.  The \"Delay\" control is used as the time delay between processing each element.  The \"Repeat/Hold\" control is used to display the message for a given time after it has completely dissolved in."
          n244 = property on="Array" class="Arr (strict)"() -> ("Number of Columns"=w360:u32)  [unwired: 2 in, 2 out]
          n245 = Array Size(array=w355) -> (size(s)=w359:i32)
          n246 = To Long Integer(number=w360) -> (32bit integer=w356:i32)
          n247 = Subtract(x=w356, y=w359) -> (x-y=w357:i32)
          n248 = Greater Than 0?(x=w357) -> (x > 0?=w358:bool)
          n249 = case shown="True" w358 {
            tunnel: w357 -> [_ w390]
            tunnel: w355 -> [_ w388]
            frame False {
              n250 = call "Too Many Characters.vi"() -> ()  [unwired: 12 in]
            }
            frame True {
              # "Playlist Shuffler (http://decibel.ni.com/content/docs/DOC-13704):"
              n251 = Divide(x=w390, y=u32 2) -> (x/y=w387:dbl)
              n252 = Round Toward -Infinity(1:w387) -> (0:w386:dbl)
              n253 = To Long Integer(number=w386) -> (32bit integer=w384:i32)
              n254 = for "#25" {
                N: w384 -> [_]
                shift-right: [w445] -> w383
                shift-left: i32[] [] -> [w447]
                n255 = Build Array (concatenate)(w447, i16 0 ("width (-)")) -> (w445:i32[])
              }
              n256 = Insert Into Array(array=w388, index=0, new element=w383) -> (w379:i32[])
              n257 = local read "Array"() -> (w380:bool[][])
              n258 = Transpose 2D Array(2D array=w380) -> (transposed array=w378:bool[][])
              n259 = for "#26" {
                shift-right: [w443] -> w381
                shift-left: w378 -> [w442]
                tunnel: w379 -> [w441] mode=indexing
                i -> [w440]
                n260 = Number To Boolean Array(number=w441) -> (Boolean array=w444:bool[])
                n261 = Insert Into Array(array=w442, index (row)=w440, new element=w444) -> (w443:bool[][])  [unwired: 1 in]
              }
              n262 = Transpose 2D Array(2D array=w381) -> (transposed array=w364:bool[][])
              n263 = Array Size(array=w364) -> (size(s)=w377:i32[])
              n264 = Index Array(array=w377, index #1=0 ("index"), index #2=1 ("index")) -> (element #1=w374:i32, element #2=w373:i32)
              n265 = for "#27" {
                N: w374 -> [_]
                tunnel: w373 -> [w431]
                shift-right: [w428] -> w365
                shift-left: i32[][] [] -> [w429]
                tunnel: w364 -> [w427]
                i -> [w430]
                n266 = for "#28" {
                  N: w431 -> [_]
                  tunnel: w430 -> [w434]
                  shift-right: [w435] -> w428
                  shift-left: w429 -> [w436]
                  tunnel: w427 -> [w432]
                  i -> [w433]
                  n267 = Index Array(array=w432, index (row)=w434, index (col)=w433) -> (element=w439:bool)
                  n268 = Boolean To (0,1)(Boolean=w439) -> (0, 1=w438:i16)
                  n269 = Build Array(w434, w433, w438) -> (w437:i32[])
                  n270 = Build Array (concatenate)(w436, w437) -> (w435:i32[][])
                }
              }
              n271 = Array Size(array=w365) -> (size(s)=w368:i32[])
              n272 = Index Array(array=w368) -> (element=w370:i32)  [unwired: 1 in]
              n273 = Decrement(x=w370) -> (x-1=w366:i32)
              n274 = Multiply(x=3 ("y"), y=w370) -> (x*y=w367:i32)
              n275 = To Double Precision Float(number=w366) -> (double precision float=w371:dbl)
              n276 = for "#29" {
                N: w367 -> [_]
                shift-right: [w415] -> w363
                shift-left: w365 -> [w418]
                tunnel: w371 -> [w426]
                n277 = Random Number (0-1)() -> (number: 0 to 1=w425:dbl)
                n278 = Multiply(x=w426, y=w425) -> (x*y=w424:dbl)
                n279 = Random Number (0-1)() -> (number: 0 to 1=w414:dbl)
                n280 = Round To Nearest(number=w424) -> (nearest integer value=w422:dbl)
                n281 = Multiply(x=w426, y=w414) -> (x*y=w423:dbl)
                n282 = Round To Nearest(number=w423) -> (nearest integer value=w421:dbl)
                n283 = To Long Integer(number=w422) -> (32bit integer=w419:i32)
                n284 = To Long Integer(number=w421) -> (32bit integer=w420:i32)
                n285 = Delete From Array(array=w418, index (row)=w419) -> (deleted portion=w416:i32[], array with subset deleted=w417:i32[][])  [unwired: 2 in]
                n286 = Insert Into Array(array=w417, index (row)=w420, new element=w416) -> (w415:i32[][])  [unwired: 1 in]
              }
              n287 = flat-sequence {
                tunnel: w363 -> [w399]
                tunnel: [w399] -> w362
                frame #0 {
                  n288 = local read "Array"() -> (w398:bool[][])
                  n289 = Array Size(array=w398) -> (size(s)=w396:i32[])
                  n290 = Index Array(array=w396, index #1=0 ("index"), index #2=1 ("index")) -> (element #1=w393:i32, element #2=w392:i32)
                  n291 = Initialize Array(TRUE, w393, w392) -> (w391:bool[][])
                  n292 = local write "Array"(w391) -> ()
                }
              }
              n293 = for "#30" {
                tunnel: w362 -> [w411] mode=indexing
                tunnel: [w400] -> w361
                n294 = Index Array(array=w411, index #1=0 ("index"), index #2=1 ("index"), index #3=2 ("index")) -> (element #1=w407:i32, element #2=w406:i32, element #3=w403:i32)
                n295 = local read "Delay"() -> (w401:u32)
                n296 = case shown="0, Default" w403 {
                  tunnel: [FALSE TRUE] -> w402
                  frame 0, Default {
                  }
                  frame 1 {
                  }
                }
                n297 = Wait (ms)(milliseconds to wait=w401) -> ()  [unwired: 1 out]
                n298 = local read "Array"() -> (w408:bool[][])
                n299 = local read "Repeat/Hold"() -> (w400:u64)
                n300 = Replace Array Subset(array=w408, new element=w402, index (row)=w407, index (col)=w406) -> (w404:bool[][])
                n301 = local write "Array"(w404) -> ()
              }
              n302 = Wait (ms)(milliseconds to wait=w361) -> ()  [unwired: 1 out]
            }
          }
        }
        frame "Dissolve Out (8)" {
          # "The number of columns that will be required to display the message is compared with the number of columns in the moving message board display based on the user's array size input.  If there are not enough columns in the display, the FALSE case presents a message to the user.  Otherwise, the TRUE case runs, which first attmepts to center the text in the display by using a for loop (#31) to pad the message with empty columns.  A second for loop (#31) is used to convert each integer value into a 1-dimensional Boolean array representing one column of the display.  The 2-dimensional Boolean array representing the display is constructed.  The message is displayed, and the \"Repeat/Hold\" control is used to display it for a given time before it starts to dissolve out.  The size of the 2-dimensional Boolean array is determined and this is used by two for loops (#33 and #34) to creat a 2-dimensional integer array with the following three pieces of information for each element of the 2-dimensioan Boolean array: row index, column index, state (0 if off/FALSE or 1 if on/TRUE).  The next for loop (#35) and the code in front of it are from here: http://decibel.ni.com/content/docs/DOC-13704, and are used to randomize the 2-dimensional integer array.  The last for loop (#36) uses the randomized 2-dimensional integer array to turn each LED element off one at a time.  The \"Delay\" control is used as the time delay between processing each element."
          n303 = property on="Array" class="Arr (strict)"() -> ("Number of Columns"=w453:u32)  [unwired: 2 in, 2 out]
          n304 = Array Size(array=w448) -> (size(s)=w452:i32)
          n305 = To Long Integer(number=w453) -> (32bit integer=w449:i32)
          n306 = Subtract(x=w449, y=w452) -> (x-y=w450:i32)
          n307 = Greater Than 0?(x=w450) -> (x > 0?=w451:bool)
          n308 = case shown="True" w451 {
            tunnel: w450 -> [_ w483]
            tunnel: w448 -> [_ w481]
            frame False {
              n309 = call "Too Many Characters.vi"() -> ()  [unwired: 12 in]
            }
            frame True {
              # "Playlist Shuffler (http://decibel.ni.com/content/docs/DOC-13704):"
              n310 = Divide(x=w483, y=u32 2) -> (x/y=w480:dbl)
              n311 = Round Toward -Infinity(1:w480) -> (0:w479:dbl)
              n312 = To Long Integer(number=w479) -> (32bit integer=w477:i32)
              n313 = for "#31" {
                N: w477 -> [_]
                shift-right: [w526] -> w476
                shift-left: i32[] [] -> [w528]
                n314 = Build Array (concatenate)(w528, i16 0 ("width (-)")) -> (w526:i32[])
              }
              n315 = Insert Into Array(array=w481, index=0, new element=w476) -> (w472:i32[])
              n316 = local read "Array"() -> (w473:bool[][])
              n317 = Transpose 2D Array(2D array=w473) -> (transposed array=w471:bool[][])
              n318 = for "#32" {
                shift-right: [w524] -> w474
                shift-left: w471 -> [w523]
                tunnel: w472 -> [w522] mode=indexing
                i -> [w521]
                n319 = Number To Boolean Array(number=w522) -> (Boolean array=w525:bool[])
                n320 = Insert Into Array(array=w523, index (row)=w521, new element=w525) -> (w524:bool[][])  [unwired: 1 in]
              }
              n321 = Transpose 2D Array(2D array=w474) -> (transposed array=w455:bool[][])
              n322 = flat-sequence {
                tunnel: [w484] -> w454
                tunnel: [w484] -> w456
                tunnel: w455 -> [w484]
                frame #0 {
                  n323 = local read "Repeat/Hold"() -> (w485:u64)
                  n324 = local write "Array"(w484) -> ()
                  n325 = Wait (ms)(milliseconds to wait=w485) -> ()  [unwired: 1 out]
                }
              }
              n326 = Array Size(array=w454) -> (size(s)=w470:i32[])
              n327 = Index Array(array=w470, index #1=0 ("index"), index #2=1 ("index")) -> (element #1=w467:i32, element #2=w466:i32)
              n328 = for "#33" {
                N: w467 -> [_]
                tunnel: w466 -> [w512]
                shift-right: [w509] -> w458
                shift-left: i32[][] [] -> [w510]
                tunnel: w456 -> [w508]
                i -> [w511]
                n329 = for "#34" {
                  N: w512 -> [_]
                  tunnel: w511 -> [w515]
                  shift-right: [w516] -> w509
                  shift-left: w510 -> [w517]
                  tunnel: w508 -> [w513]
                  i -> [w514]
                  n330 = Index Array(array=w513, index (row)=w515, index (col)=w514) -> (element=w520:bool)
                  n331 = Boolean To (0,1)(Boolean=w520) -> (0, 1=w519:i16)
                  n332 = Build Array(w515, w514, w519) -> (w518:i32[])
                  n333 = Build Array (concatenate)(w517, w518) -> (w516:i32[][])
                }
              }
              n334 = Array Size(array=w458) -> (size(s)=w461:i32[])
              n335 = Index Array(array=w461) -> (element=w463:i32)  [unwired: 1 in]
              n336 = Decrement(x=w463) -> (x-1=w459:i32)
              n337 = Multiply(x=3 ("y"), y=w463) -> (x*y=w460:i32)
              n338 = To Double Precision Float(number=w459) -> (double precision float=w464:dbl)
              n339 = for "#35" {
                N: w460 -> [_]
                shift-right: [w496] -> w457
                shift-left: w458 -> [w499]
                tunnel: w464 -> [w507]
                n340 = Random Number (0-1)() -> (number: 0 to 1=w506:dbl)
                n341 = Multiply(x=w507, y=w506) -> (x*y=w505:dbl)
                n342 = Random Number (0-1)() -> (number: 0 to 1=w495:dbl)
                n343 = Round To Nearest(number=w505) -> (nearest integer value=w503:dbl)
                n344 = Multiply(x=w507, y=w495) -> (x*y=w504:dbl)
                n345 = Round To Nearest(number=w504) -> (nearest integer value=w502:dbl)
                n346 = To Long Integer(number=w503) -> (32bit integer=w500:i32)
                n347 = To Long Integer(number=w502) -> (32bit integer=w501:i32)
                n348 = Delete From Array(array=w499, index (row)=w500) -> (deleted portion=w497:i32[], array with subset deleted=w498:i32[][])  [unwired: 2 in]
                n349 = Insert Into Array(array=w498, index (row)=w501, new element=w497) -> (w496:i32[][])  [unwired: 1 in]
              }
              n350 = for "#36" {
                tunnel: w457 -> [w494] mode=indexing
                n351 = Index Array(array=w494, index #1=0 ("index"), index #2=1 ("index")) -> (element #1=w490:i32, element #2=w489:i32)
                n352 = local read "Delay"() -> (w487:u32)
                n353 = Wait (ms)(milliseconds to wait=w487) -> ()  [unwired: 1 out]
                n354 = local read "Array"() -> (w491:bool[][])
                n355 = Replace Array Subset(array=w491, new element=FALSE, index (row)=w490, index (col)=w489) -> (w488:bool[][])
                n356 = local write "Array"(w488) -> ()
              }
            }
          }
        }
        frame "Random Pattern (9)" {
          # "The outer for loop (#37) is used to control the number of random patterns which will be displayed as disired by the user (from the \"Repeat/Hold\" control).  The inner for loops (#38 and #39) are used to create a 2-dimensional array of Booleans (based on the size of the array as specified by the user) with each element randomly selected as being on or off.  The \"Delay\" time is used as the time to wait before displaying the next random pattern."
          n357 = local read "Repeat/Hold"() -> (w531:u64)
          n358 = property on="Array" class="Arr (strict)"() -> ("Number of Rows"=w530:u32, "Number of Columns"=w529:u32)  [unwired: 2 in, 2 out]
          n359 = for "#37" {
            N: w531 -> [_]
            tunnel: w530 -> [w533]
            tunnel: w529 -> [w532]
            n360 = for "#38" {
              N: w533 -> [_]
              tunnel: [w537] -> w534 mode=indexing
              tunnel: w532 -> [w536]
              n361 = for "#39" {
                N: w536 -> [_]
                tunnel: [w538] -> w537 mode=indexing
                n362 = Random Number (0-1)() -> (number: 0 to 1=w541:dbl)
                n363 = Round To Nearest(number=w541) -> (nearest integer value=w539:dbl)
                n364 = Type Cast(type=FALSE, x=w539) -> (*(type *) &x=w538:bool)
              }
            }
            n365 = local read "Delay"() -> (w535:u32)
            n366 = Wait (ms)(milliseconds to wait=w535) -> ()  [unwired: 1 out]
            n367 = local write "Array"(w534) -> ()
          }
        }
      }
    }
    frame Error {
      n368 = call "Too Big.vi"() -> ()  [unwired: 12 in]
    }
  }
